vi "impulse_filter.vi"(6 "Reset":bool, 11 "Signal in":sgl[][](array[numeric])) -> (0 "RMS mismatch":sgl, 1 "Repair count":i32, 3 "Signal out":sgl[][](array[numeric]))   [LabVIEW 2013]
panel:
  in  "Display every":u32=1
  out "Repair count (latched)":i32
  in  "Impulse end threshold":sgl=0.001
  out "Criterion":sgl[](graph)
  out "Repaired":sgl[][](graph)
  out "Delta":sgl[][](graph)
  in  "Impulse start threshold":sgl=0.005
  # "Thresholds and RMS are approximately in volts.  See code comment for details on distance metric."
  # "Number of samples repaired"
  # "RMS difference between this block\nand the previous (all samples)."
  # "Impulse filter for PSD signals.   The rows are PSD channels, columns are time samples.   We compare the current data block to preceding blocks to see if there is significant amplitude change.   Corrupted samples are replaced with the corresponding sample from a preceding block.    We also compute an average amplitude change value across all samples."
  # "These displays have to be enabled in the block diagram."
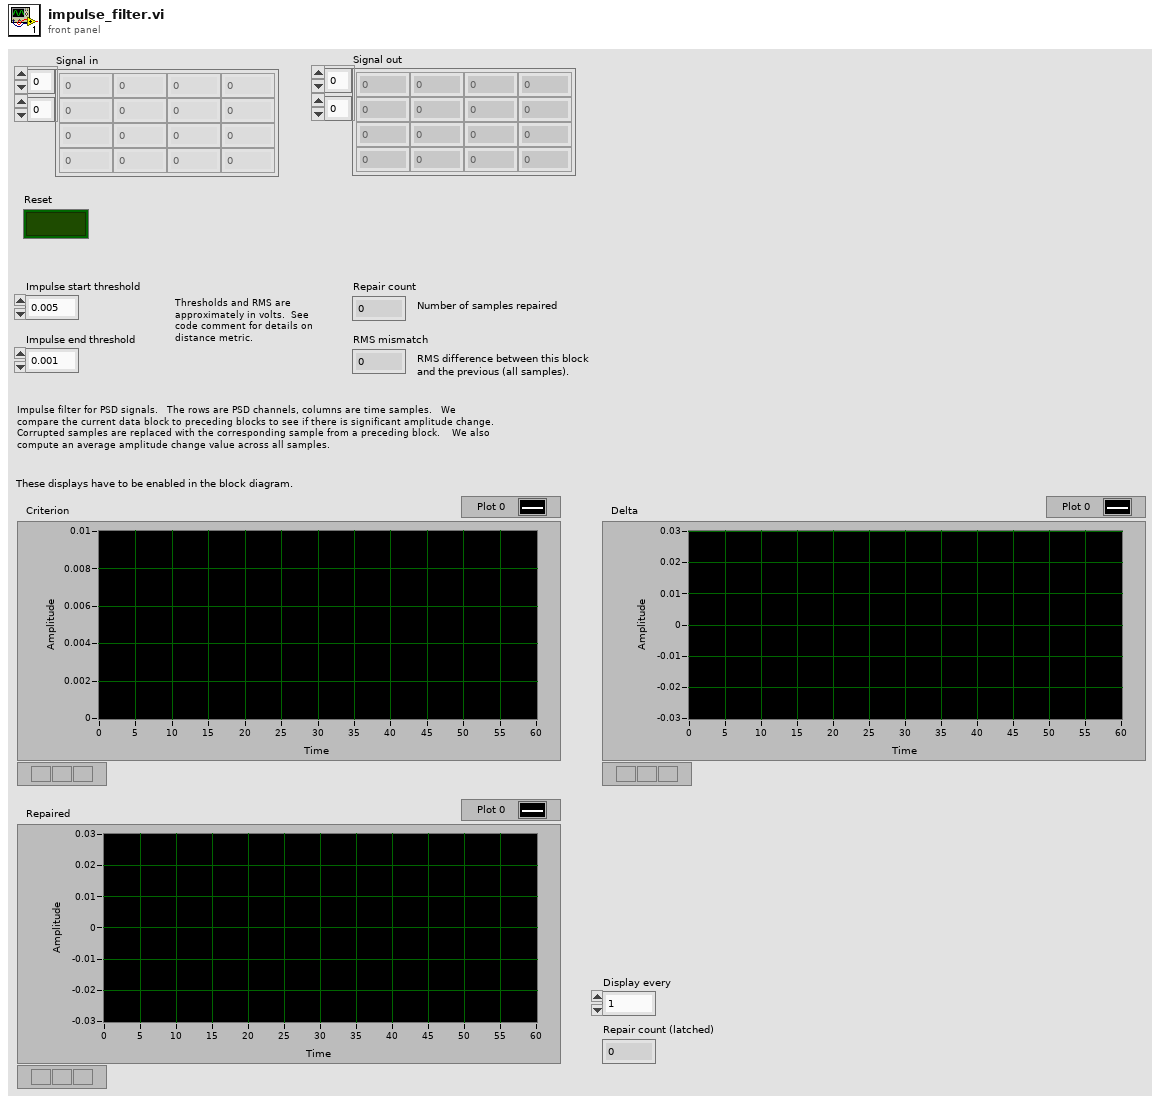
[diagram p1: front panel]
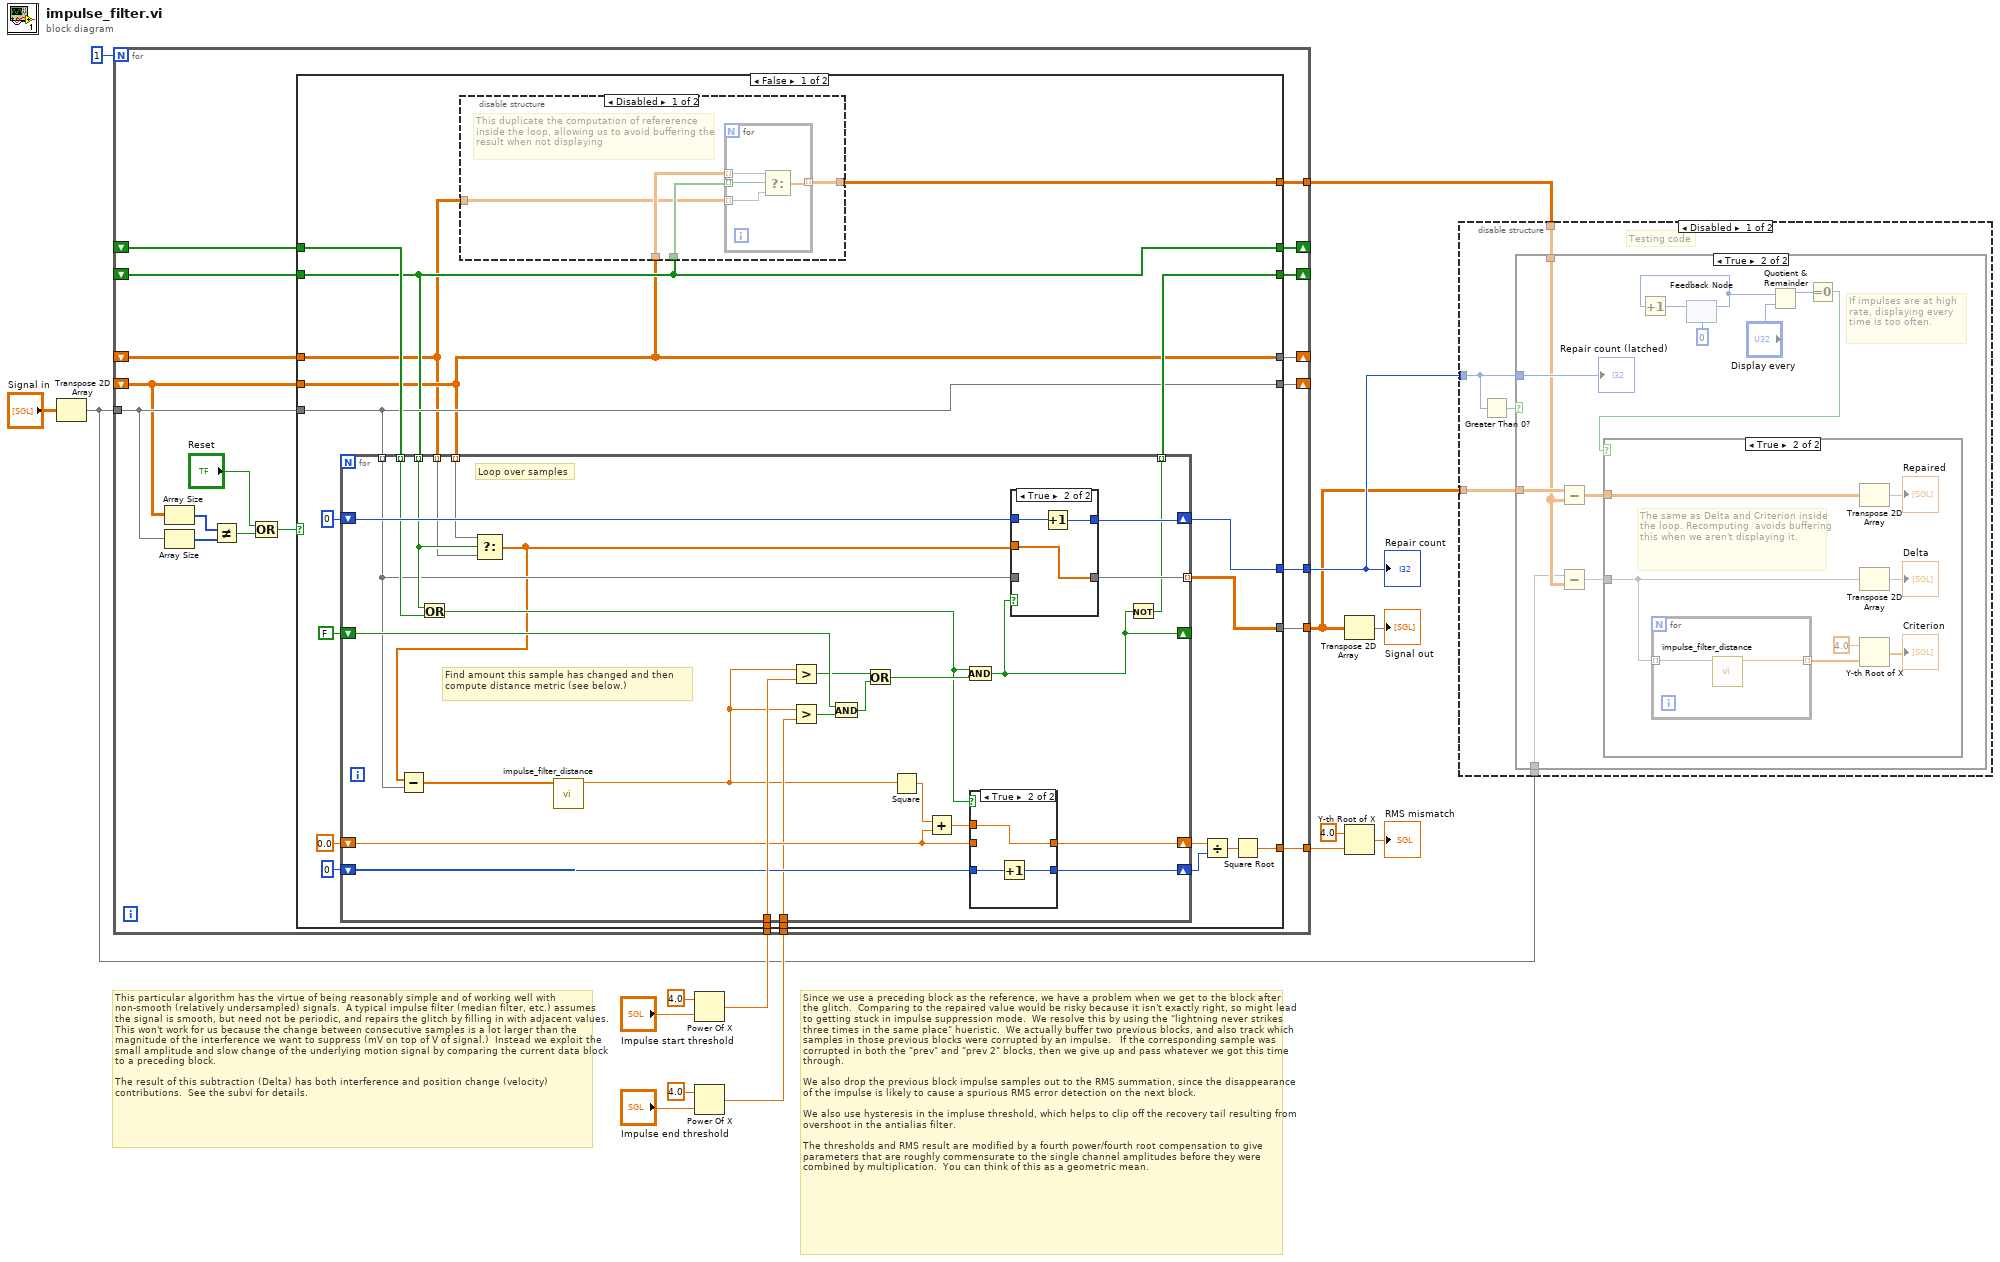
[diagram p0: block diagram]
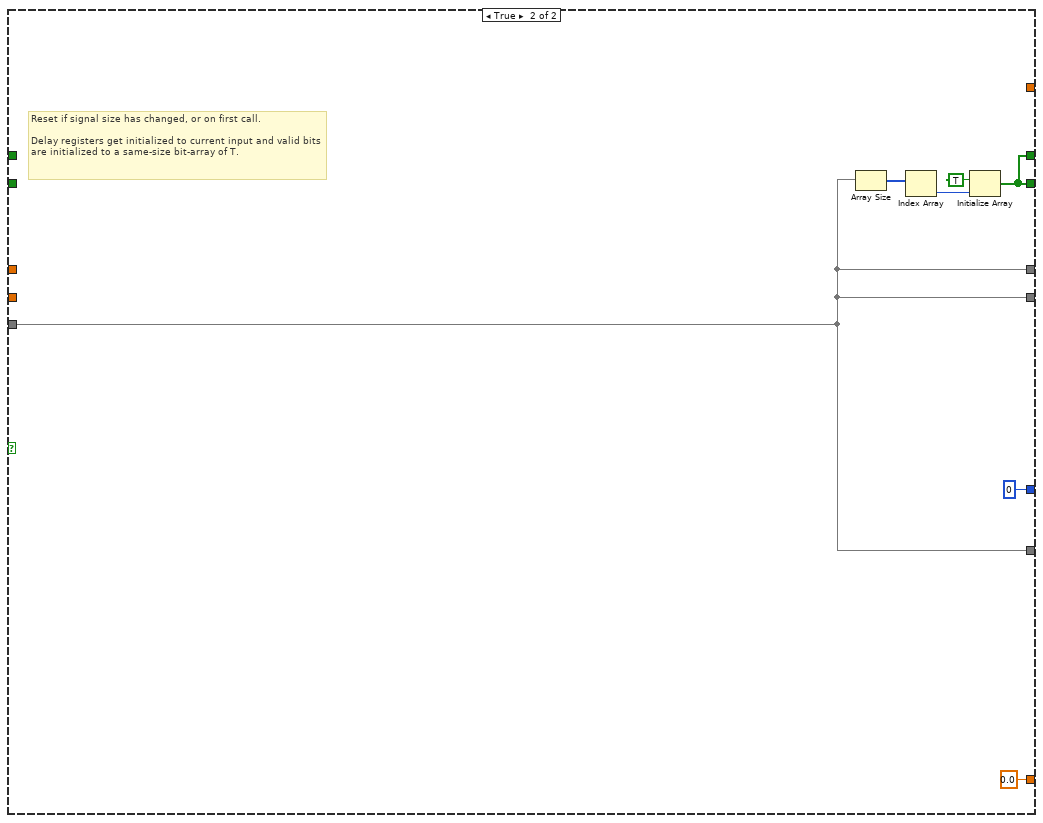
[diagram p8: hidden frame]
diagram:
  # "Since we use a preceding block as the reference, we have a problem when we get to the block after the glitch.  Comparing to the repaired value would be risky because it isn't exactly right, so might lead to getting stuck in impulse suppression mode.  We resolve this by using the \"lightning never strikes three times in the same place\" hueristic.  We actually buffer two previous blocks, and also track which samples in those previous blocks were corrupted by an impulse.   If the corresponding sample was corrupted in both the \"prev\" and \"prev 2\" blocks, then we give up and pass whatever we got this time through.\n\nWe also drop the previous block impulse samples out to the RMS summation, since the disappearance of the impulse is likely to cause a spurious RMS error detection on the next block.\n\nWe also use hysteresis in the impluse threshold, which helps to clip off the recovery tail resulting from overshoot in the antialias filter.\n\nThe thresholds and RMS result are modified by a fourth power/fourth root compensation to give parameters that are roughly commensurate to the single channel amplitudes before they were combined by multiplication.  You can think of this as a geometric mean."
  # "This particular algorithm has the virtue of being reasonably simple and of working well with non-smooth (relatively undersampled) signals.  A typical impulse filter (median filter, etc.) assumes the signal is smooth, but need not be periodic, and repairs the glitch by filling in with adjacent values.   This won't work for us because the change between consecutive samples is a lot larger than the magnitude of the interference we want to suppress (mV on top of V of signal.)  Instead we exploit the small amplitude and slow change of the underlying motion signal by comparing the current data block to a preceding block.   \n\nThe result of this subtraction (Delta) has both interference and position change (velocity) contributions.  See the subvi for details."
  n1 = Transpose 2D Array(2D array="Signal in") -> (transposed array=w1:sgl[][])
  n2 = Power Of X(1:"Impulse start threshold", 2:sgl 4.0 ("x")) -> (0:w14:sgl)
  n3 = Power Of X(1:"Impulse end threshold", 2:sgl 4.0 ("x")) -> (0:w6:sgl)
  n4 = for {
    N: 1 -> [_]
    shift-right: [w19] -> _
    shift-left: _ -> [w23]
    tunnel: w1 -> [w28]
    shift-right: [w35] -> _
    shift-left: _ -> [w22]
    tunnel: w14 -> [w34]
    tunnel: [w33] -> w2
    tunnel: [w32] -> w5
    tunnel: [w30] -> w13
    tunnel: [w18] -> w15
    tunnel: w6 -> [w29]
    shift-right: [w20] -> _
    shift-left: _ -> [w27]
    shift-right: [w26] -> _
    shift-left: _ -> [w21]
    n5 = Array Size(array=w23) -> (size(s)=w36:i32[])
    n6 = Array Size(array=w28) -> (size(s)=w31:i32[])
    n7 = Not Equal?(x=w36, y=w31) -> (x != y?=w25:bool)
    n8 = Compound Arithmetic op=OR("Reset", w25) -> (w24:bool)
    n9 = case shown="False" w24 {
      tunnel: w23 -> [w39 _]
      tunnel: w28 -> [w41 w101]
      tunnel: [w54 w102] -> w35
      tunnel: w34 -> [w55 _]
      tunnel: [w43 w101] -> w33
      tunnel: [w52 0] -> w32
      tunnel: [w48 sgl 0.0] -> w30
      tunnel: w29 -> [w44 _]
      tunnel: w27 -> [w38 _]
      tunnel: [w40 w102] -> w26
      tunnel: w22 -> [w40 _]
      tunnel: w21 -> [w42 _]
      tunnel: [w39 w101] -> w20
      tunnel: [w41 w101] -> w19
      tunnel: [w37 _] -> w18
      frame False {
        n10 = for {
          tunnel: w39 -> [w69] mode=indexing
          tunnel: w41 -> [w67] mode=indexing
          tunnel: w40 -> [w70] mode=indexing
          tunnel: w55 -> [w90]
          tunnel: [w73] -> w54 mode=indexing
          tunnel: [w82] -> w43 mode=indexing
          shift-right: [w89] -> w52
          shift-left: 0 -> [w88]
          shift-right: [w86] -> w50
          shift-left: sgl 0.0 ("sum") -> [w83]
          shift-right: [w84] -> w46
          shift-left: 0 -> [w85]
          shift-right: [w66] -> _
          shift-left: FALSE -> [w77]
          tunnel: w44 -> [w79]
          tunnel: w42 -> [w72] mode=indexing
          tunnel: w38 -> [w68] mode=indexing
          # "Find amount this sample has changed and then compute distance metric (see below.)"
          # "Loop over samples"
          n11 = Or(x=w70, y=w72) -> (x .or. y?=w71:bool)
          n12 = Select(t=w69, s=w70, f=w68) -> (s? t:f=w64:sgl[])
          n13 = Subtract(x=w64, y=w67) -> (x-y=w80:sgl[])
          n14 = call "impulse_filter_distance.vi"("Delta"=w80) -> ("Distance"=w65:sgl)  [unwired: 10 in]
          n15 = Greater?(x=w65, y=w90) -> (0:w75:bool)
          n16 = Greater?(x=w65, y=w79) -> (0:w78:bool)
          n17 = And(x=w77, y=w78) -> (x .and. y?=w74:bool)
          n18 = Or(x=w75, y=w74) -> (x .or. y?=w76:bool)
          n19 = Square(x=w65) -> (x^2=w81:sgl)
          n20 = Add(x=w81, y=w83) -> (x+y=w87:sgl)
          n21 = And(x=w71, y=w76) -> (x .and. y?=w66:bool)
          n22 = case shown="True" w71 {
            tunnel: w87 -> [_ w95]
            tunnel: [w92 w95] -> w86
            tunnel: w85 -> [w91 w94]
            tunnel: [w91 w93] -> w84
            tunnel: w83 -> [w92 _]
            frame False {
            }
            frame True {
              n23 = Increment(x=w94) -> (x+1=w93:i32)
            }
          }
          n24 = case shown="True" w66 {
            tunnel: w64 -> [_ w100]
            tunnel: w67 -> [w96 _]
            tunnel: [w96 w100] -> w82
            tunnel: [w97 w99] -> w89
            tunnel: w88 -> [w97 w98]
            frame False {
            }
            frame True {
              n25 = Increment(x=w98) -> (x+1=w99:i32)
            }
          }
          n26 = Not(x=w66) -> (.not. x?=w73:bool)
        }
        n27 = disable-structure shown="Disabled" {
          disable-tunnel: w40 -> [w59 _]
          disable-tunnel: w39 -> [w58 _]
          disable-tunnel: w38 -> [w57 _]
          disable-tunnel: [w56 _] -> w37
          frame Disabled {
            # "This duplicate the computation of refererence inside the loop, allowing us to avoid buffering the result when not displaying"
            n28 = for {
              tunnel: w59 -> [w63] mode=indexing
              tunnel: w58 -> [w62] mode=indexing
              tunnel: w57 -> [w61] mode=indexing
              tunnel: [w60] -> w56 mode=indexing
              n29 = Select(t=w62, s=w63, f=w61) -> (s? t:f=w60:sgl[])
            }
          }
          frame Enabled {
          }
        }
        n30 = Divide(x=w50, y=w46) -> (x/y=w49:sgl)
        n31 = Square Root(x=w49) -> (sqrt(x)=w48:sgl)
      }
      frame True {
        # "Reset if signal size has changed, or on first call.\n\nDelay registers get initialized to current input and valid bits are initialized to a same-size bit-array of T."
        n32 = Array Size(array=w101) -> (size(s)=w104:i32[])
        n33 = Index Array(array=w104) -> (element=w103:i32)  [unwired: 1 in]
        n34 = Initialize Array(TRUE ("x = y?"), w103) -> (w102:bool[])
      }
    }
  }
  "Repair count" <- w5
  n35 = Transpose 2D Array(2D array=w2) -> (transposed array=→"Signal out":sgl[][])
  n36 = Y-th Root of X(1:w13, 2:sgl 4.0 ("y")) -> (0:→"RMS mismatch":sgl)
  n37 = disable-structure shown="Disabled" {
    disable-tunnel: w1 -> [w111 _]
    disable-tunnel: w15 -> [w110 _]
    disable-tunnel: w5 -> [w109 _]
    disable-tunnel: w2 -> [w108 _]
    frame Disabled {
      # "Testing code"
      n38 = Greater Than 0?(x=w109) -> (x > 0?=w112:bool)
      n39 = case shown="True" w112 {
        tunnel: w111 -> [_ w115]
        tunnel: w110 -> [_ w116]
        tunnel: w109 -> [_ w119]
        tunnel: w108 -> [_ w118]
        frame False {
        }
        frame True {
          # "If impulses are at high rate, displaying every\ntime is too often."
          n40 = Subtract(x=w118, y=w116) -> (x-y=w117:sgl[][])
          n41 = Subtract(x=w115, y=w116) -> (x-y=w113:sgl[][])
          n42 = feedback #1(u32 0) -> (w122:u32)
          n43 = Increment(x=w122) -> (x+1=w123:u32)
          n44 = feedback-in #1(w123) -> ()
          n45 = Quotient & Remainder(x=w122, y="Display every") -> (x-y*floor(x/y)=w120:u32)  [unwired: 1 out]
          n46 = Equal To 0?(x=w120) -> (x = 0?=w114:bool)
          n47 = case shown="True" w114 {
            tunnel: w113 -> [_ w126]
            tunnel: w117 -> [_ w129]
            frame False {
            }
            frame True {
              # "The same as Delta and Criterion inside the loop. Recomputing  avoids buffering this when we aren't displaying it."
              n48 = for {
                tunnel: w126 -> [w133] mode=indexing
                tunnel: [w132] -> w125 mode=indexing
                n49 = call "impulse_filter_distance.vi"("Delta"=w133) -> ("Distance"=w132:sgl)  [unwired: 10 in]
              }
              n50 = Transpose 2D Array(2D array=w129) -> (transposed array=→"Repaired":sgl[][])
              n51 = Transpose 2D Array(2D array=w126) -> (transposed array=→"Delta":sgl[][])
              n52 = Y-th Root of X(1:w125, 2:sgl 4.0 ("y")) -> (0:→"Criterion":sgl[])
            }
          }
          "Repair count (latched)" <- w119
        }
      }
    }
    frame Enabled {
    }
  }
